vi "catch.vi"() -> ()   [LabVIEW 2019]
uses:
  labview project/V3_WSC_project/WSCbot_V3_Toolkit.lvlibp/WSCBOTV3_Toolkit/IO/LowLevel/PulseCounter.ctl
  labview project/V3_WSC_project/WSCbot_V3_Toolkit.lvlibp
panel:
  out "F710 button info.RB":bool
  out "Stop Output":bool
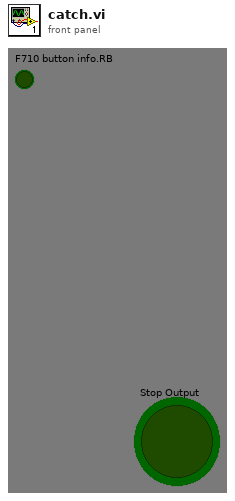
[diagram p1: front panel]
types:
  T1 = typedef "WSCbot_V3_Toolkit.lvlibp/PulseCounter.ctl" = enum16{"CH1", "CH2", "CH3", "CH4", "CH5"}
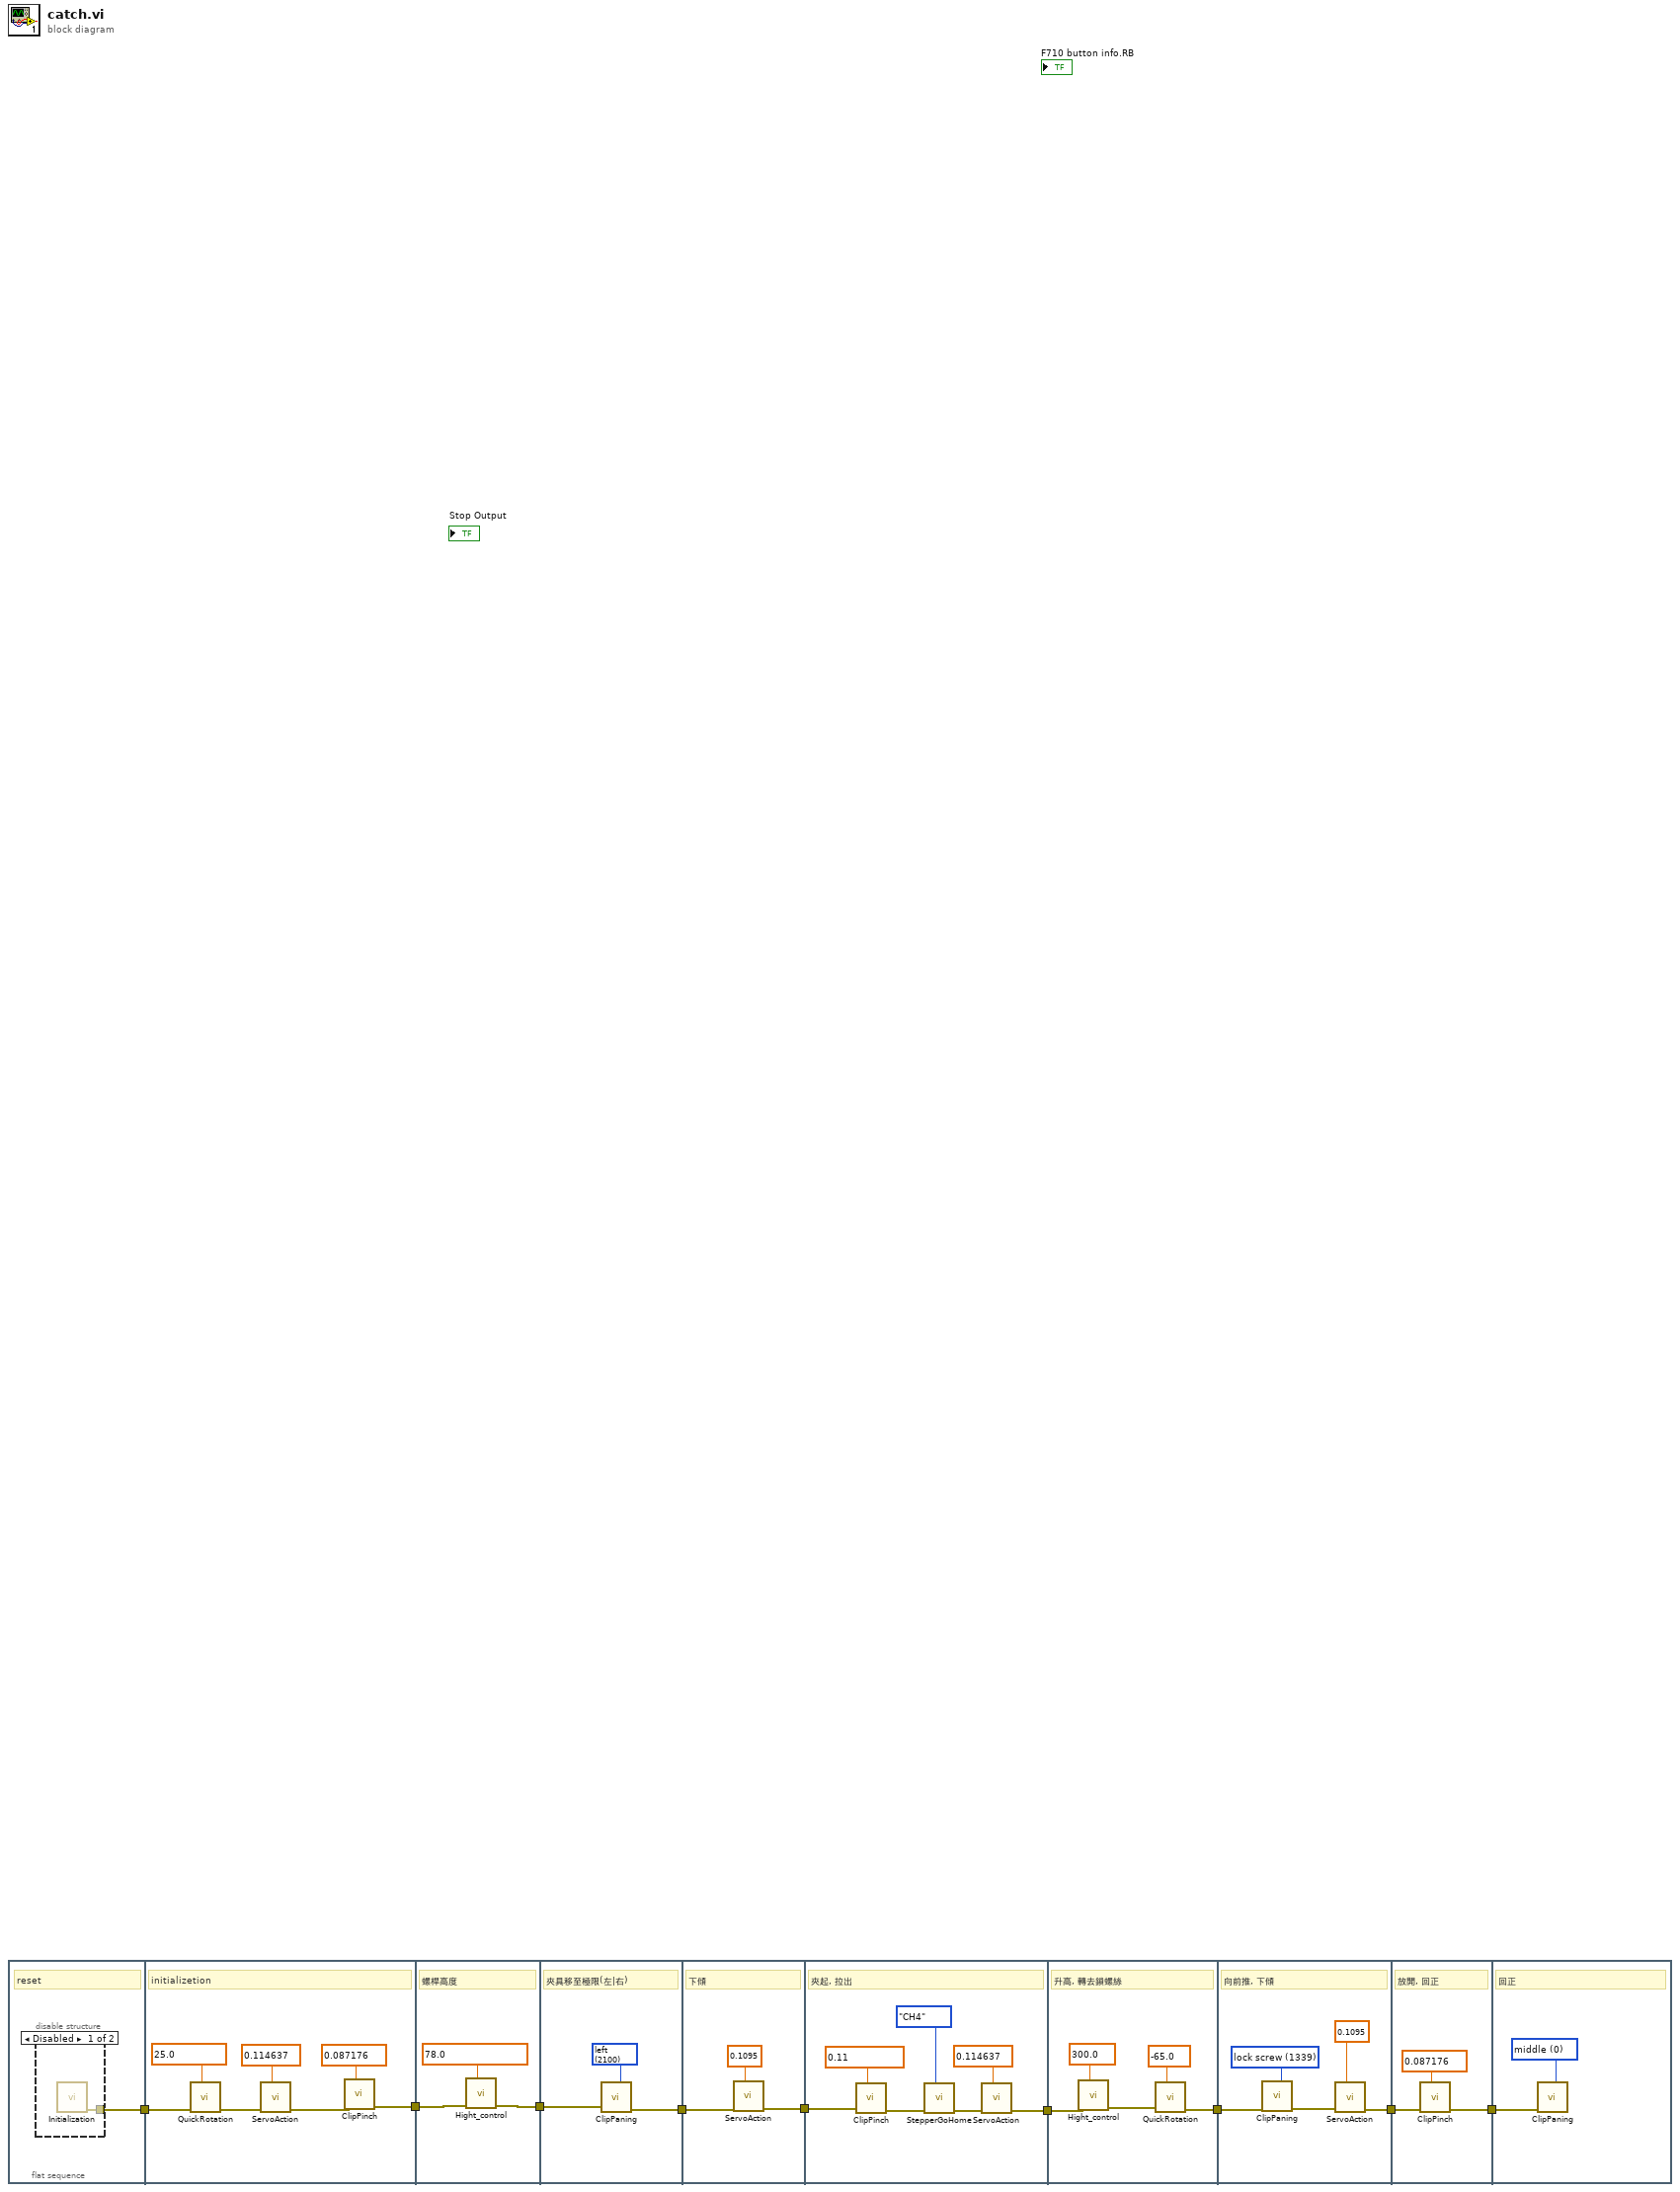
[diagram p0: block diagram]
diagram:
  n1 = flat-sequence {
    tunnel: [w10] -> w9
    tunnel: [w15] -> w7
    tunnel: w9 -> [w14]
    tunnel: w7 -> [w21]
    tunnel: [w20] -> w6
    tunnel: w6 -> [w23]
    tunnel: [w24] -> w8
    tunnel: w8 -> [w26]
    tunnel: [w27] -> w2
    tunnel: [w29] -> w5
    tunnel: w2 -> [w31]
    tunnel: w5 -> [w38]
    tunnel: [w35] -> w4
    tunnel: w4 -> [w44]
    tunnel: [w40] -> w3
    tunnel: w3 -> [w47]
    tunnel: [w45] -> w1
    tunnel: w1 -> [w48]
    frame #0 {
      # "reset"
      n2 = disable-structure shown="Disabled" {
        disable-tunnel: [w11 _] -> w10
        frame Disabled {
          n3 = call "Initialization.vi"() -> ("Error Out"=w11:errorcluster)  [unwired: 11 in]
        }
        frame Enabled {
        }
      }
    }
    frame #1 {
      w12 = 25.0 items=["Forward"=25.0, "Right"=115.0, "Left"=-65.0] ("螺桿面向")
      w17 = 0.087176 items=["pinch_up"=0.11, "release"=0.087176] ("pinch?")
      w18 = 0.114637 items=["up"=0.1095, "up_up"=0.114637, "down"=0.073446, "back"=0.037435, "back_back"=0.035] ("face_dir")
      # "initializetion"
      n4 = call "QuickRotation.vi"("螺桿面向"=w12, "Error In"=w14) -> ("Error Out"=w13:errorcluster)  [unwired: 9 in]
      n5 = call "ServoAction.vi"("face_dir"=w18, "Error In"=w13) -> ("Error Out"=w16:errorcluster)  [unwired: 9 in]
      n6 = call "ClipPinch.vi"("pinch?"=w17, "Error In"=w16) -> ("Error Out"=w15:errorcluster)  [unwired: 9 in]
    }
    frame #2 {
      w19 = 78.0 items=["最低物料櫃"=0.0, "物料櫃第二格"=78.0, "Á³´U"=138.0, "螺帽瞄準"=250.0, "最高"=300.0] ("Text Ring")
      # "螺桿高度"
      n7 = call "Hight_control.vi"("Text Ring"=w19, "Error In"=w21) -> ("Error Out"=w20:errorcluster)  [unwired: 9 in]
    }
    frame #3 {
      w22 = 2100 items=["left"=2100, "right"=-3500, "lock screw"=1339, "middle"=0] ("location")
      # "夾具移至極限(左|右)"
      n8 = call "ClipPaning.vi"("Error In"=w23, "location"=w22) -> ("Error Out"=w24:errorcluster)  [unwired: 8 in]
    }
    frame #4 {
      w25 = 0.1095 items=["up"=0.1095, "up_up"=0.114637, "down"=0.073446, "back"=0.037435, "back_back"=0.035] ("face_dir")
      # "下傾"
      n9 = call "ServoAction.vi"("face_dir"=w25, "Error In"=w26) -> ("Error Out"=w27:errorcluster)  [unwired: 9 in]
    }
    frame #5 {
      w28 = 0.114637 items=["up"=0.1095, "up_up"=0.114637, "down"=0.073446, "back"=0.037435, "back_back"=0.035] ("face_dir")
      w34 = 0.11 items=["pinch_up"=0.11, "release"=0.087176] ("pinch?")
      # "夾起, 拉出"
      n10 = call "ClipPinch.vi"("pinch?"=w34, "Error In"=w31) -> ("Error Out"=w33:errorcluster)  [unwired: 9 in]
      n11 = call "StepperGoHome.vi"("PulseCounterChanel"=PulseCounter."CH4", "Error In"=w33) -> ("Error Out"=w30:errorcluster)  [unwired: 7 in, 2 out]
      n12 = call "ServoAction.vi"("face_dir"=w28, "Error In"=w30) -> ("Error Out"=w29:errorcluster)  [unwired: 9 in]
    }
    frame #6 {
      w36 = 300.0 items=["最低物料櫃"=0.0, "物料櫃第二格"=78.0, "Á³´U"=138.0, "螺帽瞄準"=250.0, "最高"=300.0] ("Text Ring")
      w39 = -65.0 items=["Forward"=25.0, "Right"=115.0, "Left"=-65.0] ("螺桿面向")
      # "升高, 轉去鎖螺絲"
      n13 = call "Hight_control.vi"("Text Ring"=w36, "Error In"=w38) -> ("Error Out"=w37:errorcluster)  [unwired: 9 in]
      n14 = call "QuickRotation.vi"("螺桿面向"=w39, "Error In"=w37) -> ("Error Out"=w35:errorcluster)  [unwired: 9 in]
    }
    frame #7 {
      w41 = 0.1095 items=["up"=0.1095, "up_up"=0.114637, "down"=0.073446, "back"=0.037435, "back_back"=0.035] ("face_dir")
      w43 = 1339 items=["left"=2100, "right"=-3500, "lock screw"=1339, "middle"=0] ("location")
      # "向前推, 下傾"
      n15 = call "ClipPaning.vi"("Error In"=w44, "location"=w43) -> ("Error Out"=w42:errorcluster)  [unwired: 8 in]
      n16 = call "ServoAction.vi"("face_dir"=w41, "Error In"=w42) -> ("Error Out"=w40:errorcluster)  [unwired: 9 in]
    }
    frame #8 {
      w46 = 0.087176 items=["pinch_up"=0.11, "release"=0.087176] ("pinch?")
      # "放開, 回正"
      n17 = call "ClipPinch.vi"("pinch?"=w46, "Error In"=w47) -> ("Error Out"=w45:errorcluster)  [unwired: 9 in]
    }
    frame #9 {
      w49 = 0 items=["left"=2100, "right"=-3500, "lock screw"=1339, "middle"=0] ("location")
      # "回正"
      n18 = call "ClipPaning.vi"("Error In"=w48, "location"=w49) -> ()  [unwired: 8 in, 1 out]
    }
  }
